vi "Shoot_Global.vi"() -> ()   [LabVIEW 2025]
panel:
  out "SetKd":dbl=1e-06 format="%#_9g"
  out "SetKi":dbl=4.0 format="%#_9g"
  out "SetKp":dbl=1.3 format="%#_9g"
  out "SetKn":dbl=0.0001731601731602 format="%#_9g"
  out "SetRPMTarg":dbl
  out "PIDMotorOut":dbl
  out "PIDIsAuto":bool
  out "SetPIDAuto":bool
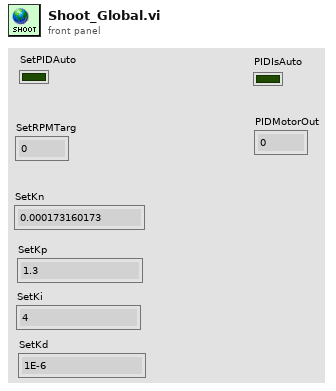
[diagram p1: front panel]
diagram:
